vi "main(Test DQMH modules).vi"() -> ()   [LabVIEW 2018, in "Application.lvlib"] (continued)
        n2572 = Replace Array Subset(array=w5988, new element=w5987) -> (w5986:bool[])  [unwired: 1 in]
        n2573 = To Variant(anything=T3."mux10_1_channel3" ("mux10_1(x6)_encode")) -> (Variant=w6003:variant)
        n2574 = To Variant(anything=T4."demux1_10_channel3" ("demux1_10(x6)_encode")) -> (Variant=w5999:variant)
        n2575 = To Variant(anything=w5986) -> (Variant=w5995:variant)
        n2576 = Bundle By Name(cluster=w5992, "command"="MEAS.mux10-1", "data"=w6003) -> (w5998:T9)
        n2577 = Bundle By Name(cluster=w5992, "command"="MEAS.demux1-10", "data"=w5999) -> (w5997:T9)
        n2578 = Bundle By Name(cluster=w5992, "command"="MEAS.eMIC", "data"=w5995) -> (w5994:T9)
        n2579 = Build Array(w5998, w5997, w5994) -> (w6021:T9[])
        n2580 = Reverse 1D Array(array=w6021) -> (reversed array=w6020:T9[])
        n2581 = for {
          tunnel: w6020 -> [w6069] mode=indexing
          tunnel: [w6066] -> w6028 mode=indexing
          tunnel: w6022 -> [w6065]
          tunnel: w6025 -> [w6070]
          n2582 = Unbundle By Name(w6069) -> ("command"=w6068:string, "data"=w6067:variant)
          n2583 = call "App enquece.vi"("Priority Enquece"=TRUE, "error in (no error)"=w6065, "command data"=w6067, "command"=w6068, "queue in"=w6070) -> ("error out"=w6066:errorcluster)  [unwired: 5 in, 1 out]
        }
        n2584 = Merge Errors(w6031, w6028) -> (w6032:errorcluster)
      }
      frame "Test Channel 4D" {
        w6077 = T9 {"command"="", "data"=variant} ("element")
        w6098 = T9 {"command"="", "data"=variant} ("element")
        w6119 = 4  # DUT channel (1-10)
        n2585 = disable-structure shown="LOGGING==TRUE" {
          disable-tunnel: w6114 -> [w6146 _]
          frame condition #0 (active) {
            n2586 = Empty String/Path?(string/path=w6146) -> (empty?=w6148:bool)
            n2587 = Select(t="Quece timeout", s=w6148, f=w6146) -> (s? t:f=w6145:string)
            n2588 = call "string log (SubVI).vi"("state Name"=w6145) -> ()  [unwired: 9 in, 2 out]
          }
          frame condition #1 {
          }
        }
        n2589 = Bundle By Name(cluster=w6098, "command"="Apps.WaitForEvent") -> (w6096:T9)
        n2590 = Bundle By Name(cluster=w6098, "command"="Apps.UI Update", "data"="D") -> (w6097:T9)
        n2591 = Bundle By Name(cluster=w6098, "command"="MEAS.AllRelaysOFF2") -> (w6091:T9)
        n2592 = Build Array(w6097, w6091, w6096) -> (w6103:T9[])
        n2593 = for {
          tunnel: [w6136] -> w6109 mode=indexing
          shift-right: [w6137] -> w6111
          shift-left: w6104 -> [w6135]
          tunnel: w6103 -> [w6134] mode=indexing
          n2594 = Unbundle By Name(w6134) -> ("command"=w6133:string, "data"=w6132:variant)
          n2595 = call "App enquece.vi"("Priority Enquece"=TRUE, "command data"=w6132, "command"=w6133, "queue in"=w6135) -> ("error out"=w6136:errorcluster, "Queue out"=w6137:refnum<queue>)  [unwired: 6 in]
        }
        n2596 = call "FGV DRV stand.vi"() -> ("Sub-Test.DCV"=w6092:bool)  [unwired: 10 in, 1 out]
        n2597 = case shown="True" w6092 {
          tunnel: [w6122 w6131] -> w6112
          frame False {
            n2598 = Build Array("WaitFor", "MEAS.requestAC") -> (w6122:string[])
          }
          frame True {
            n2599 = Build Array("Test DRV 19", "Test DRV 20", "Test DRV 21", "Test DRV 22", "WaitForD", "MEAS.requestAC") -> (w6131:string[])
          }
        }
        n2600 = Merge Errors(w6109) -> (w6102:errorcluster)
        n2601 = Reverse 1D Array(array=w6112) -> (reversed array=w6090:string[])
        n2602 = for {
          tunnel: w6090 -> [w6143] mode=indexing
          tunnel: [w6142] -> w6108 mode=indexing
          shift-right: [w6141] -> w6110
          shift-left: w6111 -> [w6144]
          tunnel: w6102 -> [w6140]
          n2603 = call "App enquece.vi"("Priority Enquece"=TRUE, "error in (no error)"=w6140, "command"=w6143, "queue in"=w6144) -> ("error out"=w6142:errorcluster, "Queue out"=w6141:refnum<queue>)  [unwired: 6 in]
        }
        n2604 = Initialize Array(FALSE ("element"), 6 ("dimension size")) -> (w6073:bool[])
        n2605 = Initialize Array(TRUE, 4 ("dimension size")) -> (w6072:bool[])
        n2606 = Merge Errors(w6108) -> (w6107:errorcluster)
        n2607 = Replace Array Subset(array=w6073, new element=w6072) -> (w6071:bool[])  [unwired: 1 in]
        n2608 = To Variant(anything=T3."mux10_1_channel4" ("mux10_1(x6)_encode")) -> (Variant=w6088:variant)
        n2609 = To Variant(anything=T4."demux1_10_channel4" ("demux1_10(x6)_encode")) -> (Variant=w6084:variant)
        n2610 = To Variant(anything=w6071) -> (Variant=w6080:variant)
        n2611 = Bundle By Name(cluster=w6077, "command"="MEAS.mux10-1", "data"=w6088) -> (w6083:T9)
        n2612 = Bundle By Name(cluster=w6077, "command"="MEAS.demux1-10", "data"=w6084) -> (w6082:T9)
        n2613 = Bundle By Name(cluster=w6077, "command"="MEAS.eMIC", "data"=w6080) -> (w6079:T9)
        n2614 = Build Array(w6083, w6082, w6079) -> (w6106:T9[])
        n2615 = Reverse 1D Array(array=w6106) -> (reversed array=w6105:T9[])
        n2616 = for {
          tunnel: w6105 -> [w6154] mode=indexing
          tunnel: [w6151] -> w6113 mode=indexing
          tunnel: w6107 -> [w6150]
          tunnel: w6110 -> [w6155]
          n2617 = Unbundle By Name(w6154) -> ("command"=w6153:string, "data"=w6152:variant)
          n2618 = call "App enquece.vi"("Priority Enquece"=TRUE, "error in (no error)"=w6150, "command data"=w6152, "command"=w6153, "queue in"=w6155) -> ("error out"=w6151:errorcluster)  [unwired: 5 in, 1 out]
        }
        n2619 = Merge Errors(w6116, w6113) -> (w6117:errorcluster)
      }
      frame "Test Channel 5D" {
        w6162 = T9 {"command"="", "data"=variant} ("element")
        w6183 = T9 {"command"="", "data"=variant} ("element")
        w6204 = 5  # DUT channel (1-10)
        n2620 = disable-structure shown="LOGGING==TRUE" {
          disable-tunnel: w6199 -> [w6231 _]
          frame condition #0 (active) {
            n2621 = Empty String/Path?(string/path=w6231) -> (empty?=w6233:bool)
            n2622 = Select(t="Quece timeout", s=w6233, f=w6231) -> (s? t:f=w6230:string)
            n2623 = call "string log (SubVI).vi"("state Name"=w6230) -> ()  [unwired: 9 in, 2 out]
          }
          frame condition #1 {
          }
        }
        n2624 = Bundle By Name(cluster=w6183, "command"="Apps.UI Update", "data"="D") -> (w6182:T9)
        n2625 = Bundle By Name(cluster=w6183, "command"="MEAS.AllRelaysOFF2") -> (w6176:T9)
        n2626 = Bundle By Name(cluster=w6183, "command"="Apps.WaitForEvent") -> (w6181:T9)
        n2627 = Build Array(w6182, w6176, w6181) -> (w6188:T9[])
        n2628 = for {
          tunnel: [w6221] -> w6194 mode=indexing
          shift-right: [w6222] -> w6196
          shift-left: w6189 -> [w6220]
          tunnel: w6188 -> [w6219] mode=indexing
          n2629 = Unbundle By Name(w6219) -> ("command"=w6218:string, "data"=w6217:variant)
          n2630 = call "App enquece.vi"("Priority Enquece"=TRUE, "command data"=w6217, "command"=w6218, "queue in"=w6220) -> ("error out"=w6221:errorcluster, "Queue out"=w6222:refnum<queue>)  [unwired: 6 in]
        }
        n2631 = call "FGV DRV stand.vi"() -> ("Sub-Test.DCV"=w6177:bool)  [unwired: 10 in, 1 out]
        n2632 = case shown="True" w6177 {
          tunnel: [w6207 w6216] -> w6197
          frame False {
            n2633 = Build Array("WaitFor", "MEAS.requestAC") -> (w6207:string[])
          }
          frame True {
            n2634 = Build Array("Test DRV 25", "Test DRV 26", "Test DRV 27", "Test DRV 28", "WaitForD", "MEAS.requestAC") -> (w6216:string[])
          }
        }
        n2635 = Merge Errors(w6194) -> (w6187:errorcluster)
        n2636 = Reverse 1D Array(array=w6197) -> (reversed array=w6175:string[])
        n2637 = for {
          tunnel: w6175 -> [w6228] mode=indexing
          tunnel: [w6227] -> w6193 mode=indexing
          shift-right: [w6226] -> w6195
          shift-left: w6196 -> [w6229]
          tunnel: w6187 -> [w6225]
          n2638 = call "App enquece.vi"("Priority Enquece"=TRUE, "error in (no error)"=w6225, "command"=w6228, "queue in"=w6229) -> ("error out"=w6227:errorcluster, "Queue out"=w6226:refnum<queue>)  [unwired: 6 in]
        }
        n2639 = Merge Errors(w6193) -> (w6192:errorcluster)
        n2640 = Initialize Array(FALSE ("element"), 6 ("dimension size")) -> (w6158:bool[])
        n2641 = Initialize Array(TRUE, 4 ("dimension size")) -> (w6157:bool[])
        n2642 = Replace Array Subset(array=w6158, new element=w6157) -> (w6156:bool[])  [unwired: 1 in]
        n2643 = To Variant(anything=T3."mux10_1_channel5" ("mux10_1(x6)_encode")) -> (Variant=w6173:variant)
        n2644 = To Variant(anything=T4."demux1_10_channel5" ("demux1_10(x6)_encode")) -> (Variant=w6169:variant)
        n2645 = To Variant(anything=w6156) -> (Variant=w6165:variant)
        n2646 = Bundle By Name(cluster=w6162, "command"="MEAS.mux10-1", "data"=w6173) -> (w6168:T9)
        n2647 = Bundle By Name(cluster=w6162, "command"="MEAS.demux1-10", "data"=w6169) -> (w6167:T9)
        n2648 = Bundle By Name(cluster=w6162, "command"="MEAS.eMIC", "data"=w6165) -> (w6164:T9)
        n2649 = Build Array(w6168, w6167, w6164) -> (w6191:T9[])
        n2650 = Reverse 1D Array(array=w6191) -> (reversed array=w6190:T9[])
        n2651 = for {
          tunnel: w6190 -> [w6239] mode=indexing
          tunnel: [w6236] -> w6198 mode=indexing
          tunnel: w6192 -> [w6235]
          tunnel: w6195 -> [w6240]
          n2652 = Unbundle By Name(w6239) -> ("command"=w6238:string, "data"=w6237:variant)
          n2653 = call "App enquece.vi"("Priority Enquece"=TRUE, "error in (no error)"=w6235, "command data"=w6237, "command"=w6238, "queue in"=w6240) -> ("error out"=w6236:errorcluster)  [unwired: 5 in, 1 out]
        }
        n2654 = Merge Errors(w6201, w6198) -> (w6202:errorcluster)
      }
      frame "Test Channel 6D" {
        w6247 = T9 {"command"="", "data"=variant} ("element")
        w6268 = T9 {"command"="", "data"=variant} ("element")
        w6289 = 6  # DUT channel (1-10)
        n2655 = disable-structure shown="LOGGING==TRUE" {
          disable-tunnel: w6284 -> [w6316 _]
          frame condition #0 (active) {
            n2656 = Empty String/Path?(string/path=w6316) -> (empty?=w6318:bool)
            n2657 = Select(t="Quece timeout", s=w6318, f=w6316) -> (s? t:f=w6315:string)
            n2658 = call "string log (SubVI).vi"("state Name"=w6315) -> ()  [unwired: 9 in, 2 out]
          }
          frame condition #1 {
          }
        }
        n2659 = Bundle By Name(cluster=w6268, "command"="Apps.UI Update", "data"="D") -> (w6267:T9)
        n2660 = Bundle By Name(cluster=w6268, "command"="MEAS.AllRelaysOFF2") -> (w6261:T9)
        n2661 = Bundle By Name(cluster=w6268, "command"="Apps.WaitForEvent") -> (w6266:T9)
        n2662 = Build Array(w6267, w6261, w6266) -> (w6273:T9[])
        n2663 = for {
          tunnel: [w6306] -> w6279 mode=indexing
          shift-right: [w6307] -> w6281
          shift-left: w6274 -> [w6305]
          tunnel: w6273 -> [w6304] mode=indexing
          n2664 = Unbundle By Name(w6304) -> ("command"=w6303:string, "data"=w6302:variant)
          n2665 = call "App enquece.vi"("Priority Enquece"=TRUE, "command data"=w6302, "command"=w6303, "queue in"=w6305) -> ("error out"=w6306:errorcluster, "Queue out"=w6307:refnum<queue>)  [unwired: 6 in]
        }
        n2666 = call "FGV DRV stand.vi"() -> ("Sub-Test.DCV"=w6262:bool)  [unwired: 10 in, 1 out]
        n2667 = case shown="True" w6262 {
          tunnel: [w6292 w6301] -> w6282
          frame False {
            n2668 = Build Array("WaitFor", "MEAS.requestAC") -> (w6292:string[])
          }
          frame True {
            n2669 = Build Array("Test DRV 31", "Test DRV 32", "Test DRV 33", "Test DRV 34", "WaitForD", "MEAS.requestAC") -> (w6301:string[])
          }
        }
        n2670 = Merge Errors(w6279) -> (w6272:errorcluster)
        n2671 = Reverse 1D Array(array=w6282) -> (reversed array=w6260:string[])
        n2672 = for {
          tunnel: w6260 -> [w6313] mode=indexing
          tunnel: [w6312] -> w6278 mode=indexing
          shift-right: [w6311] -> w6280
          shift-left: w6281 -> [w6314]
          tunnel: w6272 -> [w6310]
          n2673 = call "App enquece.vi"("Priority Enquece"=TRUE, "error in (no error)"=w6310, "command"=w6313, "queue in"=w6314) -> ("error out"=w6312:errorcluster, "Queue out"=w6311:refnum<queue>)  [unwired: 6 in]
        }
        n2674 = Initialize Array(FALSE ("element"), 6 ("dimension size")) -> (w6243:bool[])
        n2675 = Initialize Array(TRUE, 4 ("dimension size")) -> (w6242:bool[])
        n2676 = Merge Errors(w6278) -> (w6277:errorcluster)
        n2677 = Replace Array Subset(array=w6243, new element=w6242) -> (w6241:bool[])  [unwired: 1 in]
        n2678 = To Variant(anything=T3."mux10_1_channel6" ("mux10_1(x6)_encode")) -> (Variant=w6258:variant)
        n2679 = To Variant(anything=T4."demux1_10_channel6" ("demux1_10(x6)_encode")) -> (Variant=w6254:variant)
        n2680 = To Variant(anything=w6241) -> (Variant=w6250:variant)
        n2681 = Bundle By Name(cluster=w6247, "command"="MEAS.mux10-1", "data"=w6258) -> (w6253:T9)
        n2682 = Bundle By Name(cluster=w6247, "command"="MEAS.demux1-10", "data"=w6254) -> (w6252:T9)
        n2683 = Bundle By Name(cluster=w6247, "command"="MEAS.eMIC", "data"=w6250) -> (w6249:T9)
        n2684 = Build Array(w6253, w6252, w6249) -> (w6276:T9[])
        n2685 = Reverse 1D Array(array=w6276) -> (reversed array=w6275:T9[])
        n2686 = for {
          tunnel: w6275 -> [w6324] mode=indexing
          tunnel: [w6321] -> w6283 mode=indexing
          tunnel: w6277 -> [w6320]
          tunnel: w6280 -> [w6325]
          n2687 = Unbundle By Name(w6324) -> ("command"=w6323:string, "data"=w6322:variant)
          n2688 = call "App enquece.vi"("Priority Enquece"=TRUE, "error in (no error)"=w6320, "command data"=w6322, "command"=w6323, "queue in"=w6325) -> ("error out"=w6321:errorcluster)  [unwired: 5 in, 1 out]
        }
        n2689 = Merge Errors(w6286, w6283) -> (w6287:errorcluster)
      }
      frame "Test Channel 7D" {
        w6332 = T9 {"command"="", "data"=variant} ("element")
        w6353 = T9 {"command"="", "data"=variant} ("element")
        w6374 = 7  # DUT channel (1-10)
        n2690 = disable-structure shown="LOGGING==TRUE" {
          disable-tunnel: w6369 -> [w6401 _]
          frame condition #0 (active) {
            n2691 = Empty String/Path?(string/path=w6401) -> (empty?=w6403:bool)
            n2692 = Select(t="Quece timeout", s=w6403, f=w6401) -> (s? t:f=w6400:string)
            n2693 = call "string log (SubVI).vi"("state Name"=w6400) -> ()  [unwired: 9 in, 2 out]
          }
          frame condition #1 {
          }
        }
        n2694 = Bundle By Name(cluster=w6353, "command"="Apps.UI Update", "data"="D") -> (w6352:T9)
        n2695 = Bundle By Name(cluster=w6353, "command"="MEAS.AllRelaysOFF2") -> (w6346:T9)
        n2696 = Bundle By Name(cluster=w6353, "command"="Apps.WaitForEvent") -> (w6351:T9)
        n2697 = Build Array(w6352, w6346, w6351) -> (w6358:T9[])
        n2698 = for {
          tunnel: [w6391] -> w6364 mode=indexing
          shift-right: [w6392] -> w6366
          shift-left: w6359 -> [w6390]
          tunnel: w6358 -> [w6389] mode=indexing
          n2699 = Unbundle By Name(w6389) -> ("command"=w6388:string, "data"=w6387:variant)
          n2700 = call "App enquece.vi"("Priority Enquece"=TRUE, "command data"=w6387, "command"=w6388, "queue in"=w6390) -> ("error out"=w6391:errorcluster, "Queue out"=w6392:refnum<queue>)  [unwired: 6 in]
        }
        n2701 = call "FGV DRV stand.vi"() -> ("Sub-Test.DCV"=w6347:bool)  [unwired: 10 in, 1 out]
        n2702 = case shown="True" w6347 {
          tunnel: [w6377 w6386] -> w6367
          frame False {
            n2703 = Build Array("WaitFor", "MEAS.requestAC") -> (w6377:string[])
          }
          frame True {
            n2704 = Build Array("Test DRV 37", "Test DRV 38", "Test DRV 39", "Test DRV 40", "WaitForD", "MEAS.requestAC") -> (w6386:string[])
          }
        }
        n2705 = Merge Errors(w6364) -> (w6357:errorcluster)
        n2706 = Reverse 1D Array(array=w6367) -> (reversed array=w6345:string[])
        n2707 = for {
          tunnel: w6345 -> [w6398] mode=indexing
          tunnel: [w6397] -> w6363 mode=indexing
          shift-right: [w6396] -> w6365
          shift-left: w6366 -> [w6399]
          tunnel: w6357 -> [w6395]
          n2708 = call "App enquece.vi"("Priority Enquece"=TRUE, "error in (no error)"=w6395, "command"=w6398, "queue in"=w6399) -> ("error out"=w6397:errorcluster, "Queue out"=w6396:refnum<queue>)  [unwired: 6 in]
        }
        n2709 = Initialize Array(FALSE ("element"), 6 ("dimension size")) -> (w6328:bool[])
        n2710 = Initialize Array(TRUE, 4 ("dimension size")) -> (w6327:bool[])
        n2711 = Merge Errors(w6363) -> (w6362:errorcluster)
        n2712 = Replace Array Subset(array=w6328, new element=w6327) -> (w6326:bool[])  [unwired: 1 in]
        n2713 = To Variant(anything=T3."mux10_1_channel7" ("mux10_1(x6)_encode")) -> (Variant=w6343:variant)
        n2714 = To Variant(anything=T4."demux1_10_channel7" ("demux1_10(x6)_encode")) -> (Variant=w6339:variant)
        n2715 = To Variant(anything=w6326) -> (Variant=w6335:variant)
        n2716 = Bundle By Name(cluster=w6332, "command"="MEAS.mux10-1", "data"=w6343) -> (w6338:T9)
        n2717 = Bundle By Name(cluster=w6332, "command"="MEAS.demux1-10", "data"=w6339) -> (w6337:T9)
        n2718 = Bundle By Name(cluster=w6332, "command"="MEAS.eMIC", "data"=w6335) -> (w6334:T9)
        n2719 = Build Array(w6338, w6337, w6334) -> (w6361:T9[])
        n2720 = Reverse 1D Array(array=w6361) -> (reversed array=w6360:T9[])
        n2721 = for {
          tunnel: w6360 -> [w6409] mode=indexing
          tunnel: [w6406] -> w6368 mode=indexing
          tunnel: w6362 -> [w6405]
          tunnel: w6365 -> [w6410]
          n2722 = Unbundle By Name(w6409) -> ("command"=w6408:string, "data"=w6407:variant)
          n2723 = call "App enquece.vi"("Priority Enquece"=TRUE, "error in (no error)"=w6405, "command data"=w6407, "command"=w6408, "queue in"=w6410) -> ("error out"=w6406:errorcluster)  [unwired: 5 in, 1 out]
        }
        n2724 = Merge Errors(w6371, w6368) -> (w6372:errorcluster)
      }
      frame "Test Channel 8D" {
        w6417 = T9 {"command"="", "data"=variant} ("element")
        w6438 = T9 {"command"="", "data"=variant} ("element")
        w6459 = 8  # DUT channel (1-10)
        n2725 = disable-structure shown="LOGGING==TRUE" {
          disable-tunnel: w6454 -> [w6486 _]
          frame condition #0 (active) {
            n2726 = Empty String/Path?(string/path=w6486) -> (empty?=w6488:bool)
            n2727 = Select(t="Quece timeout", s=w6488, f=w6486) -> (s? t:f=w6485:string)
            n2728 = call "string log (SubVI).vi"("state Name"=w6485) -> ()  [unwired: 9 in, 2 out]
          }
          frame condition #1 {
          }
        }
        n2729 = Bundle By Name(cluster=w6438, "command"="Apps.UI Update", "data"="D") -> (w6437:T9)
        n2730 = Bundle By Name(cluster=w6438, "command"="MEAS.AllRelaysOFF2") -> (w6431:T9)
        n2731 = Bundle By Name(cluster=w6438, "command"="Apps.WaitForEvent") -> (w6436:T9)
        n2732 = Build Array(w6437, w6431, w6436) -> (w6443:T9[])
        n2733 = for {
          tunnel: [w6476] -> w6449 mode=indexing
          shift-right: [w6477] -> w6451
          shift-left: w6444 -> [w6475]
          tunnel: w6443 -> [w6474] mode=indexing
          n2734 = Unbundle By Name(w6474) -> ("command"=w6473:string, "data"=w6472:variant)
          n2735 = call "App enquece.vi"("Priority Enquece"=TRUE, "command data"=w6472, "command"=w6473, "queue in"=w6475) -> ("error out"=w6476:errorcluster, "Queue out"=w6477:refnum<queue>)  [unwired: 6 in]
        }
        n2736 = call "FGV DRV stand.vi"() -> ("Sub-Test.DCV"=w6432:bool)  [unwired: 10 in, 1 out]
        n2737 = case shown="True" w6432 {
          tunnel: [w6462 w6471] -> w6452
          frame False {
            n2738 = Build Array("WaitFor", "MEAS.requestAC") -> (w6462:string[])
          }
          frame True {
            n2739 = Build Array("Test DRV 43", "Test DRV 44", "Test DRV 45", "Test DRV 46", "WaitForD", "MEAS.requestAC") -> (w6471:string[])
          }
        }
        n2740 = Merge Errors(w6449) -> (w6442:errorcluster)
        n2741 = Reverse 1D Array(array=w6452) -> (reversed array=w6430:string[])
        n2742 = for {
          tunnel: w6430 -> [w6483] mode=indexing
          tunnel: [w6482] -> w6448 mode=indexing
          shift-right: [w6481] -> w6450
          shift-left: w6451 -> [w6484]
          tunnel: w6442 -> [w6480]
          n2743 = call "App enquece.vi"("Priority Enquece"=TRUE, "error in (no error)"=w6480, "command"=w6483, "queue in"=w6484) -> ("error out"=w6482:errorcluster, "Queue out"=w6481:refnum<queue>)  [unwired: 6 in]
        }
        n2744 = Initialize Array(FALSE ("element"), 6 ("dimension size")) -> (w6413:bool[])
        n2745 = Initialize Array(TRUE, 4 ("dimension size")) -> (w6412:bool[])
        n2746 = Merge Errors(w6448) -> (w6447:errorcluster)
        n2747 = Replace Array Subset(array=w6413, new element=w6412) -> (w6411:bool[])  [unwired: 1 in]
        n2748 = To Variant(anything=T3."mux10_1_channel8" ("mux10_1(x6)_encode")) -> (Variant=w6428:variant)
        n2749 = To Variant(anything=T4."demux1_10_channel8" ("demux1_10(x6)_encode")) -> (Variant=w6424:variant)
        n2750 = To Variant(anything=w6411) -> (Variant=w6420:variant)
        n2751 = Bundle By Name(cluster=w6417, "command"="MEAS.mux10-1", "data"=w6428) -> (w6423:T9)
        n2752 = Bundle By Name(cluster=w6417, "command"="MEAS.demux1-10", "data"=w6424) -> (w6422:T9)
        n2753 = Bundle By Name(cluster=w6417, "command"="MEAS.eMIC", "data"=w6420) -> (w6419:T9)
        n2754 = Build Array(w6423, w6422, w6419) -> (w6446:T9[])
        n2755 = Reverse 1D Array(array=w6446) -> (reversed array=w6445:T9[])
        n2756 = for {
          tunnel: w6445 -> [w6494] mode=indexing
          tunnel: [w6491] -> w6453 mode=indexing
          tunnel: w6447 -> [w6490]
          tunnel: w6450 -> [w6495]
          n2757 = Unbundle By Name(w6494) -> ("command"=w6493:string, "data"=w6492:variant)
          n2758 = call "App enquece.vi"("Priority Enquece"=TRUE, "error in (no error)"=w6490, "command data"=w6492, "command"=w6493, "queue in"=w6495) -> ("error out"=w6491:errorcluster)  [unwired: 5 in, 1 out]
        }
        n2759 = Merge Errors(w6456, w6453) -> (w6457:errorcluster)
      }
      frame "Test Channel 9D" {
        w6502 = T9 {"command"="", "data"=variant} ("element")
        w6523 = T9 {"command"="", "data"=variant} ("element")
        w6544 = 9  # DUT channel (1-10)
        n2760 = disable-structure shown="LOGGING==TRUE" {
          disable-tunnel: w6539 -> [w6571 _]
          frame condition #0 (active) {
            n2761 = Empty String/Path?(string/path=w6571) -> (empty?=w6573:bool)
            n2762 = Select(t="Quece timeout", s=w6573, f=w6571) -> (s? t:f=w6570:string)
            n2763 = call "string log (SubVI).vi"("state Name"=w6570) -> ()  [unwired: 9 in, 2 out]
          }
          frame condition #1 {
          }
        }
        n2764 = Bundle By Name(cluster=w6523, "command"="Apps.UI Update", "data"="D") -> (w6522:T9)
        n2765 = Bundle By Name(cluster=w6523, "command"="MEAS.AllRelaysOFF2") -> (w6516:T9)
        n2766 = Bundle By Name(cluster=w6523, "command"="Apps.WaitForEvent") -> (w6521:T9)
        n2767 = Build Array(w6522, w6516, w6521) -> (w6528:T9[])
        n2768 = for {
          tunnel: [w6561] -> w6534 mode=indexing
          shift-right: [w6562] -> w6536
          shift-left: w6529 -> [w6560]
          tunnel: w6528 -> [w6559] mode=indexing
          n2769 = Unbundle By Name(w6559) -> ("command"=w6558:string, "data"=w6557:variant)
          n2770 = call "App enquece.vi"("Priority Enquece"=TRUE, "command data"=w6557, "command"=w6558, "queue in"=w6560) -> ("error out"=w6561:errorcluster, "Queue out"=w6562:refnum<queue>)  [unwired: 6 in]
        }
        n2771 = call "FGV DRV stand.vi"() -> ("Sub-Test.DCV"=w6517:bool)  [unwired: 10 in, 1 out]
        n2772 = case shown="False" w6517 {
          tunnel: [w6547 w6556] -> w6537
          frame False {
            n2773 = Build Array("WaitFor", "MEAS.requestAC") -> (w6547:string[])
          }
          frame True {
            n2774 = Build Array("Test DRV 49", "Test DRV 50", "Test DRV 51", "Test DRV 52", "WaitForD", "MEAS.requestAC") -> (w6556:string[])
          }
        }
        n2775 = Merge Errors(w6534) -> (w6527:errorcluster)
        n2776 = Reverse 1D Array(array=w6537) -> (reversed array=w6515:string[])
        n2777 = for {
          tunnel: w6515 -> [w6568] mode=indexing
          tunnel: [w6567] -> w6533 mode=indexing
          shift-right: [w6566] -> w6535
          shift-left: w6536 -> [w6569]
          tunnel: w6527 -> [w6565]
          n2778 = call "App enquece.vi"("Priority Enquece"=TRUE, "error in (no error)"=w6565, "command"=w6568, "queue in"=w6569) -> ("error out"=w6567:errorcluster, "Queue out"=w6566:refnum<queue>)  [unwired: 6 in]
        }
        n2779 = Initialize Array(FALSE ("element"), 6 ("dimension size")) -> (w6498:bool[])
        n2780 = Initialize Array(TRUE, 4 ("dimension size")) -> (w6497:bool[])
        n2781 = Merge Errors(w6533) -> (w6532:errorcluster)
        n2782 = Replace Array Subset(array=w6498, new element=w6497) -> (w6496:bool[])  [unwired: 1 in]
        n2783 = To Variant(anything=T3."mux10_1_channel9" ("mux10_1(x6)_encode")) -> (Variant=w6513:variant)
        n2784 = To Variant(anything=T4."demux1_10_channel9" ("demux1_10(x6)_encode")) -> (Variant=w6509:variant)
        n2785 = To Variant(anything=w6496) -> (Variant=w6505:variant)
        n2786 = Bundle By Name(cluster=w6502, "command"="MEAS.mux10-1", "data"=w6513) -> (w6508:T9)
        n2787 = Bundle By Name(cluster=w6502, "command"="MEAS.demux1-10", "data"=w6509) -> (w6507:T9)
        n2788 = Bundle By Name(cluster=w6502, "command"="MEAS.eMIC", "data"=w6505) -> (w6504:T9)
        n2789 = Build Array(w6508, w6507, w6504) -> (w6531:T9[])
        n2790 = Reverse 1D Array(array=w6531) -> (reversed array=w6530:T9[])
        n2791 = for {
          tunnel: w6530 -> [w6579] mode=indexing
          tunnel: [w6576] -> w6538 mode=indexing
          tunnel: w6532 -> [w6575]
          tunnel: w6535 -> [w6580]
          n2792 = Unbundle By Name(w6579) -> ("command"=w6578:string, "data"=w6577:variant)
          n2793 = call "App enquece.vi"("Priority Enquece"=TRUE, "error in (no error)"=w6575, "command data"=w6577, "command"=w6578, "queue in"=w6580) -> ("error out"=w6576:errorcluster)  [unwired: 5 in, 1 out]
        }
        n2794 = Merge Errors(w6541, w6538) -> (w6542:errorcluster)
      }
      frame "Test Channel 10E" {
        w6587 = T9 {"command"="", "data"=variant} ("element")
        w6609 = T9 {"command"="", "data"=variant} ("element")
        w6629 = 10  # DUT channel (1-10)
        n2795 = disable-structure shown="LOGGING==TRUE" {
          disable-tunnel: w6624 -> [w6657 _]
          frame condition #0 (active) {
            n2796 = Empty String/Path?(string/path=w6657) -> (empty?=w6659:bool)
            n2797 = Select(t="Quece timeout", s=w6659, f=w6657) -> (s? t:f=w6656:string)
            n2798 = call "string log (SubVI).vi"("state Name"=w6656) -> ()  [unwired: 9 in, 2 out]
          }
          frame condition #1 {
          }
        }
        n2799 = Bundle By Name(cluster=w6609, "command"="Apps.UI Update", "data"="E") -> (w6608:T9)
        n2800 = Bundle By Name(cluster=w6609, "command"="MEAS.AllRelaysOFF2") -> (w6601:T9)
        n2801 = Bundle By Name(cluster=w6609, "command"="Apps.WaitForEvent") -> (w6607:T9)
        n2802 = Build Array(w6608, w6601, w6607) -> (w6614:T9[])
        n2803 = for {
          tunnel: [w6647] -> w6620 mode=indexing
          shift-right: [w6648] -> w6622
          shift-left: w6615 -> [w6646]
          tunnel: w6614 -> [w6645] mode=indexing
          n2804 = Unbundle By Name(w6645) -> ("command"=w6644:string, "data"=w6643:variant)
          n2805 = call "App enquece.vi"("Priority Enquece"=TRUE, "command data"=w6643, "command"=w6644, "queue in"=w6646) -> ("error out"=w6647:errorcluster, "Queue out"=w6648:refnum<queue>)  [unwired: 6 in]
        }
        n2806 = call "FGV DRV stand.vi"() -> ("Sub-Test.DCV"=w6602:bool)  [unwired: 10 in, 1 out]
        n2807 = case shown="True" w6602 {
          tunnel: [w6633 w6635] -> w6604
          frame False {
            n2808 = Build Array("WaitFor", "MEAS.requestAC") -> (w6633:string[])
          }
          frame True {
            n2809 = Build Array("Test DRV 55", "Test DRV 56", "Test DRV 57", "Test DRV 58", "Test DRV 59", "WaitForE", "MEAS.requestAC") -> (w6635:string[])
          }
        }
        n2810 = Merge Errors(w6620) -> (w6613:errorcluster)
        n2811 = Reverse 1D Array(array=w6604) -> (reversed array=w6600:string[])
        n2812 = for {
          tunnel: w6600 -> [w6654] mode=indexing
          tunnel: [w6653] -> w6619 mode=indexing
          shift-right: [w6652] -> w6621
          shift-left: w6622 -> [w6655]
          tunnel: w6613 -> [w6651]
          n2813 = call "App enquece.vi"("Priority Enquece"=TRUE, "error in (no error)"=w6651, "command"=w6654, "queue in"=w6655) -> ("error out"=w6653:errorcluster, "Queue out"=w6652:refnum<queue>)  [unwired: 6 in]
        }
        n2814 = Initialize Array(FALSE ("element"), 6 ("dimension size")) -> (w6583:bool[])
        n2815 = Initialize Array(TRUE, 5 ("dimension size")) -> (w6582:bool[])
        n2816 = Merge Errors(w6619) -> (w6618:errorcluster)
        n2817 = Replace Array Subset(array=w6583, new element=w6582) -> (w6581:bool[])  [unwired: 1 in]
        n2818 = To Variant(anything=T3."mux10_1_channel10" ("mux10_1(x6)_encode")) -> (Variant=w6598:variant)
        n2819 = To Variant(anything=T4."demux1_10_channel10" ("demux1_10(x6)_encode")) -> (Variant=w6594:variant)
        n2820 = To Variant(anything=w6581) -> (Variant=w6590:variant)
        n2821 = Bundle By Name(cluster=w6587, "command"="MEAS.mux10-1", "data"=w6598) -> (w6593:T9)
        n2822 = Bundle By Name(cluster=w6587, "command"="MEAS.demux1-10", "data"=w6594) -> (w6592:T9)
        n2823 = Bundle By Name(cluster=w6587, "command"="MEAS.eMIC", "data"=w6590) -> (w6589:T9)
        n2824 = Build Array(w6593, w6592, w6589) -> (w6617:T9[])
        n2825 = Reverse 1D Array(array=w6617) -> (reversed array=w6616:T9[])
        n2826 = for {
          tunnel: w6616 -> [w6665] mode=indexing
          tunnel: [w6662] -> w6623 mode=indexing
          tunnel: w6618 -> [w6661]
          tunnel: w6621 -> [w6666]
          n2827 = Unbundle By Name(w6665) -> ("command"=w6664:string, "data"=w6663:variant)
          n2828 = call "App enquece.vi"("Priority Enquece"=TRUE, "error in (no error)"=w6661, "command data"=w6663, "command"=w6664, "queue in"=w6666) -> ("error out"=w6662:errorcluster)  [unwired: 5 in, 1 out]
        }
        n2829 = Merge Errors(w6626, w6623) -> (w6627:errorcluster)
      }
      frame "Test Channel 1E" {
        w6673 = T9 {"command"="", "data"=variant} ("element")
        w6695 = T9 {"command"="", "data"=variant} ("element")
        w6715 = 1  # DUT channel (1-10)
        n2830 = disable-structure shown="LOGGING==TRUE" {
          disable-tunnel: w6710 -> [w6743 _]
          frame condition #0 (active) {
            n2831 = Empty String/Path?(string/path=w6743) -> (empty?=w6745:bool)
            n2832 = Select(t="Quece timeout", s=w6745, f=w6743) -> (s? t:f=w6742:string)
            n2833 = call "string log (SubVI).vi"("state Name"=w6742) -> ()  [unwired: 9 in, 2 out]
          }
          frame condition #1 {
          }
        }
        n2834 = Bundle By Name(cluster=w6695, "command"="Apps.UI Update", "data"="E") -> (w6694:T9)
        n2835 = Bundle By Name(cluster=w6695, "command"="MEAS.AllRelaysOFF2") -> (w6687:T9)
        n2836 = Bundle By Name(cluster=w6695, "command"="Apps.WaitForEvent") -> (w6693:T9)
        n2837 = Build Array(w6694, w6687, w6693) -> (w6700:T9[])
        n2838 = for {
          tunnel: [w6733] -> w6706 mode=indexing
          shift-right: [w6734] -> w6708
          shift-left: w6701 -> [w6732]
          tunnel: w6700 -> [w6731] mode=indexing
          n2839 = Unbundle By Name(w6731) -> ("command"=w6730:string, "data"=w6729:variant)
          n2840 = call "App enquece.vi"("Priority Enquece"=TRUE, "command data"=w6729, "command"=w6730, "queue in"=w6732) -> ("error out"=w6733:errorcluster, "Queue out"=w6734:refnum<queue>)  [unwired: 6 in]
        }
        n2841 = call "FGV DRV stand.vi"() -> ("Sub-Test.DCV"=w6688:bool)  [unwired: 10 in, 1 out]
        n2842 = case shown="True" w6688 {
          tunnel: [w6719 w6721] -> w6690
          frame False {
            n2843 = Build Array("WaitFor", "MEAS.requestAC") -> (w6719:string[])
          }
          frame True {
            n2844 = Build Array("Test DRV 1", "Test DRV 2", "Test DRV 3", "Test DRV 4", "Test DRV 5", "WaitForE", "MEAS.requestAC") -> (w6721:string[])
          }
        }
        n2845 = Merge Errors(w6706) -> (w6699:errorcluster)
        n2846 = Reverse 1D Array(array=w6690) -> (reversed array=w6686:string[])
        n2847 = for {
          tunnel: w6686 -> [w6740] mode=indexing
          tunnel: [w6739] -> w6705 mode=indexing
          shift-right: [w6738] -> w6707
          shift-left: w6708 -> [w6741]
          tunnel: w6699 -> [w6737]
          n2848 = call "App enquece.vi"("Priority Enquece"=TRUE, "error in (no error)"=w6737, "command"=w6740, "queue in"=w6741) -> ("error out"=w6739:errorcluster, "Queue out"=w6738:refnum<queue>)  [unwired: 6 in]
        }
        n2849 = Initialize Array(FALSE ("element"), 6 ("dimension size")) -> (w6669:bool[])
        n2850 = Initialize Array(TRUE, 5 ("dimension size")) -> (w6668:bool[])
        n2851 = Merge Errors(w6705) -> (w6704:errorcluster)
        n2852 = Replace Array Subset(array=w6669, new element=w6668) -> (w6667:bool[])  [unwired: 1 in]
        n2853 = To Variant(anything=T3."mux10_1_channel1" ("mux10_1(x6)_encode")) -> (Variant=w6684:variant)
        n2854 = To Variant(anything=T4."demux1_10_channel1" ("demux1_10(x6)_encode")) -> (Variant=w6680:variant)
        n2855 = To Variant(anything=w6667) -> (Variant=w6676:variant)
        n2856 = Bundle By Name(cluster=w6673, "command"="MEAS.mux10-1", "data"=w6684) -> (w6679:T9)
        n2857 = Bundle By Name(cluster=w6673, "command"="MEAS.demux1-10", "data"=w6680) -> (w6678:T9)
        n2858 = Bundle By Name(cluster=w6673, "command"="MEAS.eMIC", "data"=w6676) -> (w6675:T9)
        n2859 = Build Array(w6679, w6678, w6675) -> (w6703:T9[])
        n2860 = Reverse 1D Array(array=w6703) -> (reversed array=w6702:T9[])
        n2861 = for {
          tunnel: w6702 -> [w6751] mode=indexing
          tunnel: [w6748] -> w6709 mode=indexing
          tunnel: w6704 -> [w6747]
          tunnel: w6707 -> [w6752]
          n2862 = Unbundle By Name(w6751) -> ("command"=w6750:string, "data"=w6749:variant)
          n2863 = call "App enquece.vi"("Priority Enquece"=TRUE, "error in (no error)"=w6747, "command data"=w6749, "command"=w6750, "queue in"=w6752) -> ("error out"=w6748:errorcluster)  [unwired: 5 in, 1 out]
        }
        n2864 = Merge Errors(w6712, w6709) -> (w6713:errorcluster)
      }
      frame "Test Channel 2E" {
        w6759 = T9 {"command"="", "data"=variant} ("element")
        w6781 = T9 {"command"="", "data"=variant} ("element")
        w6801 = 2  # DUT channel (1-10)
        n2865 = disable-structure shown="LOGGING==TRUE" {
          disable-tunnel: w6796 -> [w6829 _]
          frame condition #0 (active) {
            n2866 = Empty String/Path?(string/path=w6829) -> (empty?=w6831:bool)
            n2867 = Select(t="Quece timeout", s=w6831, f=w6829) -> (s? t:f=w6828:string)
            n2868 = call "string log (SubVI).vi"("state Name"=w6828) -> ()  [unwired: 9 in, 2 out]
          }
          frame condition #1 {
          }
        }
        n2869 = Bundle By Name(cluster=w6781, "command"="Apps.UI Update", "data"="E") -> (w6780:T9)
        n2870 = Bundle By Name(cluster=w6781, "command"="MEAS.AllRelaysOFF2") -> (w6773:T9)
        n2871 = Bundle By Name(cluster=w6781, "command"="Apps.WaitForEvent") -> (w6779:T9)
        n2872 = Build Array(w6780, w6773, w6779) -> (w6786:T9[])
        n2873 = for {
          tunnel: [w6819] -> w6792 mode=indexing
          shift-right: [w6820] -> w6794
          shift-left: w6787 -> [w6818]
          tunnel: w6786 -> [w6817] mode=indexing
          n2874 = Unbundle By Name(w6817) -> ("command"=w6816:string, "data"=w6815:variant)
          n2875 = call "App enquece.vi"("Priority Enquece"=TRUE, "command data"=w6815, "command"=w6816, "queue in"=w6818) -> ("error out"=w6819:errorcluster, "Queue out"=w6820:refnum<queue>)  [unwired: 6 in]
        }
        n2876 = call "FGV DRV stand.vi"() -> ("Sub-Test.DCV"=w6774:bool)  [unwired: 10 in, 1 out]
        n2877 = case shown="True" w6774 {
          tunnel: [w6805 w6807] -> w6776
          frame False {
            n2878 = Build Array("WaitFor", "MEAS.requestAC") -> (w6805:string[])
          }
          frame True {
            n2879 = Build Array("Test DRV 7", "Test DRV 8", "Test DRV 9", "Test DRV 10", "Test DRV 11", "WaitForE", "MEAS.requestAC") -> (w6807:string[])
          }
        }
        n2880 = Merge Errors(w6792) -> (w6785:errorcluster)
        n2881 = Reverse 1D Array(array=w6776) -> (reversed array=w6772:string[])
        n2882 = for {
          tunnel: w6772 -> [w6826] mode=indexing
          tunnel: [w6825] -> w6791 mode=indexing
          shift-right: [w6824] -> w6793
          shift-left: w6794 -> [w6827]
          tunnel: w6785 -> [w6823]
          n2883 = call "App enquece.vi"("Priority Enquece"=TRUE, "error in (no error)"=w6823, "command"=w6826, "queue in"=w6827) -> ("error out"=w6825:errorcluster, "Queue out"=w6824:refnum<queue>)  [unwired: 6 in]
        }
        n2884 = Initialize Array(FALSE ("element"), 6 ("dimension size")) -> (w6755:bool[])
        n2885 = Initialize Array(TRUE, 5 ("dimension size")) -> (w6754:bool[])
        n2886 = Merge Errors(w6791) -> (w6790:errorcluster)
        n2887 = Replace Array Subset(array=w6755, new element=w6754) -> (w6753:bool[])  [unwired: 1 in]
        n2888 = To Variant(anything=w6753) -> (Variant=w6762:variant)
        n2889 = To Variant(anything=T3."mux10_1_channel2" ("mux10_1(x6)_encode")) -> (Variant=w6770:variant)
        n2890 = To Variant(anything=T4."demux1_10_channel2" ("demux1_10(x6)_encode")) -> (Variant=w6766:variant)
        n2891 = Bundle By Name(cluster=w6759, "command"="MEAS.mux10-1", "data"=w6770) -> (w6765:T9)
        n2892 = Bundle By Name(cluster=w6759, "command"="MEAS.demux1-10", "data"=w6766) -> (w6764:T9)
        n2893 = Bundle By Name(cluster=w6759, "command"="MEAS.eMIC", "data"=w6762) -> (w6761:T9)
        n2894 = Build Array(w6765, w6764, w6761) -> (w6789:T9[])
        n2895 = Reverse 1D Array(array=w6789) -> (reversed array=w6788:T9[])
        n2896 = for {
          tunnel: w6788 -> [w6837] mode=indexing
          tunnel: [w6834] -> w6795 mode=indexing
          tunnel: w6790 -> [w6833]
          tunnel: w6793 -> [w6838]
          n2897 = Unbundle By Name(w6837) -> ("command"=w6836:string, "data"=w6835:variant)
          n2898 = call "App enquece.vi"("Priority Enquece"=TRUE, "error in (no error)"=w6833, "command data"=w6835, "command"=w6836, "queue in"=w6838) -> ("error out"=w6834:errorcluster)  [unwired: 5 in, 1 out]
        }
        n2899 = Merge Errors(w6798, w6795) -> (w6799:errorcluster)
      }
      frame "Test Channel 3E" {
        w6845 = T9 {"command"="", "data"=variant} ("element")
        w6867 = T9 {"command"="", "data"=variant} ("element")
        w6887 = 3  # DUT channel (1-10)
        n2900 = disable-structure shown="LOGGING==TRUE" {
          disable-tunnel: w6882 -> [w6915 _]
          frame condition #0 (active) {
            n2901 = Empty String/Path?(string/path=w6915) -> (empty?=w6917:bool)
            n2902 = Select(t="Quece timeout", s=w6917, f=w6915) -> (s? t:f=w6914:string)
            n2903 = call "string log (SubVI).vi"("state Name"=w6914) -> ()  [unwired: 9 in, 2 out]
          }
          frame condition #1 {
          }
        }
        n2904 = Bundle By Name(cluster=w6867, "command"="Apps.UI Update", "data"="E") -> (w6866:T9)
        n2905 = Bundle By Name(cluster=w6867, "command"="MEAS.AllRelaysOFF2") -> (w6859:T9)
        n2906 = Bundle By Name(cluster=w6867, "command"="Apps.WaitForEvent") -> (w6865:T9)
        n2907 = Build Array(w6866, w6859, w6865) -> (w6872:T9[])
        n2908 = for {
          tunnel: [w6905] -> w6878 mode=indexing
          shift-right: [w6906] -> w6880
          shift-left: w6873 -> [w6904]
          tunnel: w6872 -> [w6903] mode=indexing
          n2909 = Unbundle By Name(w6903) -> ("command"=w6902:string, "data"=w6901:variant)
          n2910 = call "App enquece.vi"("Priority Enquece"=TRUE, "command data"=w6901, "command"=w6902, "queue in"=w6904) -> ("error out"=w6905:errorcluster, "Queue out"=w6906:refnum<queue>)  [unwired: 6 in]
        }
        n2911 = call "FGV DRV stand.vi"() -> ("Sub-Test.DCV"=w6860:bool)  [unwired: 10 in, 1 out]
        n2912 = case shown="True" w6860 {
          tunnel: [w6891 w6893] -> w6862
          frame False {
            n2913 = Build Array("WaitFor", "MEAS.requestAC") -> (w6891:string[])
          }
          frame True {
            n2914 = Build Array("Test DRV 13", "Test DRV 14", "Test DRV 15", "Test DRV 16", "Test DRV 17", "WaitForE", "MEAS.requestAC") -> (w6893:string[])
          }
        }
        n2915 = Merge Errors(w6878) -> (w6871:errorcluster)
        n2916 = Reverse 1D Array(array=w6862) -> (reversed array=w6858:string[])
        n2917 = for {
          tunnel: w6858 -> [w6912] mode=indexing
          tunnel: [w6911] -> w6877 mode=indexing
          shift-right: [w6910] -> w6879
          shift-left: w6880 -> [w6913]
          tunnel: w6871 -> [w6909]
          n2918 = call "App enquece.vi"("Priority Enquece"=TRUE, "error in (no error)"=w6909, "command"=w6912, "queue in"=w6913) -> ("error out"=w6911:errorcluster, "Queue out"=w6910:refnum<queue>)  [unwired: 6 in]
        }
        n2919 = Initialize Array(FALSE ("element"), 6 ("dimension size")) -> (w6841:bool[])
        n2920 = Initialize Array(TRUE, 5 ("dimension size")) -> (w6840:bool[])
        n2921 = Replace Array Subset(array=w6841, new element=w6840) -> (w6839:bool[])  [unwired: 1 in]
        n2922 = Merge Errors(w6877) -> (w6876:errorcluster)
        n2923 = To Variant(anything=T3."mux10_1_channel3" ("mux10_1(x6)_encode")) -> (Variant=w6856:variant)
        n2924 = To Variant(anything=T4."demux1_10_channel3" ("demux1_10(x6)_encode")) -> (Variant=w6852:variant)
        n2925 = To Variant(anything=w6839) -> (Variant=w6848:variant)
        n2926 = Bundle By Name(cluster=w6845, "command"="MEAS.mux10-1", "data"=w6856) -> (w6851:T9)
        n2927 = Bundle By Name(cluster=w6845, "command"="MEAS.demux1-10", "data"=w6852) -> (w6850:T9)
        n2928 = Bundle By Name(cluster=w6845, "command"="MEAS.eMIC", "data"=w6848) -> (w6847:T9)
        n2929 = Build Array(w6851, w6850, w6847) -> (w6875:T9[])
        n2930 = Reverse 1D Array(array=w6875) -> (reversed array=w6874:T9[])
        n2931 = for {
          tunnel: w6874 -> [w6923] mode=indexing
          tunnel: [w6920] -> w6881 mode=indexing
          tunnel: w6876 -> [w6919]
          tunnel: w6879 -> [w6924]
          n2932 = Unbundle By Name(w6923) -> ("command"=w6922:string, "data"=w6921:variant)
          n2933 = call "App enquece.vi"("Priority Enquece"=TRUE, "error in (no error)"=w6919, "command data"=w6921, "command"=w6922, "queue in"=w6924) -> ("error out"=w6920:errorcluster)  [unwired: 5 in, 1 out]
        }
        n2934 = Merge Errors(w6884, w6881) -> (w6885:errorcluster)
      }
      frame "Test Channel 4E" {
        w6931 = T9 {"command"="", "data"=variant} ("element")
        w6953 = T9 {"command"="", "data"=variant} ("element")
        w6973 = 4  # DUT channel (1-10)
        n2935 = disable-structure shown="LOGGING==TRUE" {
          disable-tunnel: w6968 -> [w7001 _]
          frame condition #0 (active) {
            n2936 = Empty String/Path?(string/path=w7001) -> (empty?=w7003:bool)
            n2937 = Select(t="Quece timeout", s=w7003, f=w7001) -> (s? t:f=w7000:string)
            n2938 = call "string log (SubVI).vi"("state Name"=w7000) -> ()  [unwired: 9 in, 2 out]
          }
          frame condition #1 {
          }
        }
        n2939 = Bundle By Name(cluster=w6953, "command"="Apps.UI Update", "data"="E") -> (w6952:T9)
        n2940 = Bundle By Name(cluster=w6953, "command"="MEAS.AllRelaysOFF2") -> (w6945:T9)
        n2941 = Bundle By Name(cluster=w6953, "command"="Apps.WaitForEvent") -> (w6951:T9)
        n2942 = Build Array(w6952, w6945, w6951) -> (w6958:T9[])
        n2943 = for {
          tunnel: [w6991] -> w6964 mode=indexing
          shift-right: [w6992] -> w6966
          shift-left: w6959 -> [w6990]
          tunnel: w6958 -> [w6989] mode=indexing
          n2944 = Unbundle By Name(w6989) -> ("command"=w6988:string, "data"=w6987:variant)
          n2945 = call "App enquece.vi"("Priority Enquece"=TRUE, "command data"=w6987, "command"=w6988, "queue in"=w6990) -> ("error out"=w6991:errorcluster, "Queue out"=w6992:refnum<queue>)  [unwired: 6 in]
        }
        n2946 = call "FGV DRV stand.vi"() -> ("Sub-Test.DCV"=w6946:bool)  [unwired: 10 in, 1 out]
        n2947 = case shown="True" w6946 {
          tunnel: [w6977 w6979] -> w6948
          frame False {
            n2948 = Build Array("WaitFor", "MEAS.requestAC") -> (w6977:string[])
          }
          frame True {
            n2949 = Build Array("Test DRV 19", "Test DRV 20", "Test DRV 21", "Test DRV 22", "Test DRV 23", "WaitForE", "MEAS.requestAC") -> (w6979:string[])
          }
        }
        n2950 = Merge Errors(w6964) -> (w6957:errorcluster)
        n2951 = Reverse 1D Array(array=w6948) -> (reversed array=w6944:string[])
        n2952 = for {
          tunnel: w6944 -> [w6998] mode=indexing
          tunnel: [w6997] -> w6963 mode=indexing
          shift-right: [w6996] -> w6965
          shift-left: w6966 -> [w6999]
          tunnel: w6957 -> [w6995]
          n2953 = call "App enquece.vi"("Priority Enquece"=TRUE, "error in (no error)"=w6995, "command"=w6998, "queue in"=w6999) -> ("error out"=w6997:errorcluster, "Queue out"=w6996:refnum<queue>)  [unwired: 6 in]
        }
        n2954 = Initialize Array(FALSE ("element"), 6 ("dimension size")) -> (w6927:bool[])
        n2955 = Initialize Array(TRUE, 5 ("dimension size")) -> (w6926:bool[])
        n2956 = Merge Errors(w6963) -> (w6962:errorcluster)
        n2957 = Replace Array Subset(array=w6927, new element=w6926) -> (w6925:bool[])  [unwired: 1 in]
        n2958 = To Variant(anything=T3."mux10_1_channel4" ("mux10_1(x6)_encode")) -> (Variant=w6942:variant)
        n2959 = To Variant(anything=T4."demux1_10_channel4" ("demux1_10(x6)_encode")) -> (Variant=w6938:variant)
        n2960 = To Variant(anything=w6925) -> (Variant=w6934:variant)
        n2961 = Bundle By Name(cluster=w6931, "command"="MEAS.mux10-1", "data"=w6942) -> (w6937:T9)
        n2962 = Bundle By Name(cluster=w6931, "command"="MEAS.demux1-10", "data"=w6938) -> (w6936:T9)
        n2963 = Bundle By Name(cluster=w6931, "command"="MEAS.eMIC", "data"=w6934) -> (w6933:T9)
        n2964 = Build Array(w6937, w6936, w6933) -> (w6961:T9[])
        n2965 = Reverse 1D Array(array=w6961) -> (reversed array=w6960:T9[])
        n2966 = for {
          tunnel: w6960 -> [w7009] mode=indexing
          tunnel: [w7006] -> w6967 mode=indexing
          tunnel: w6962 -> [w7005]
          tunnel: w6965 -> [w7010]
          n2967 = Unbundle By Name(w7009) -> ("command"=w7008:string, "data"=w7007:variant)
          n2968 = call "App enquece.vi"("Priority Enquece"=TRUE, "error in (no error)"=w7005, "command data"=w7007, "command"=w7008, "queue in"=w7010) -> ("error out"=w7006:errorcluster)  [unwired: 5 in, 1 out]
        }
        n2969 = Merge Errors(w6970, w6967) -> (w6971:errorcluster)
      }
      frame "Test Channel 5E" {
        w7017 = T9 {"command"="", "data"=variant} ("element")
        w7039 = T9 {"command"="", "data"=variant} ("element")
        w7059 = 5  # DUT channel (1-10)
        n2970 = disable-structure shown="LOGGING==TRUE" {
          disable-tunnel: w7054 -> [w7087 _]
          frame condition #0 (active) {
            n2971 = Empty String/Path?(string/path=w7087) -> (empty?=w7089:bool)
            n2972 = Select(t="Quece timeout", s=w7089, f=w7087) -> (s? t:f=w7086:string)
            n2973 = call "string log (SubVI).vi"("state Name"=w7086) -> ()  [unwired: 9 in, 2 out]
          }
          frame condition #1 {
          }
        }
        n2974 = Bundle By Name(cluster=w7039, "command"="Apps.UI Update", "data"="E") -> (w7038:T9)
        n2975 = Bundle By Name(cluster=w7039, "command"="MEAS.AllRelaysOFF2") -> (w7031:T9)
        n2976 = Bundle By Name(cluster=w7039, "command"="Apps.WaitForEvent") -> (w7037:T9)
        n2977 = Build Array(w7038, w7031, w7037) -> (w7044:T9[])
        n2978 = for {
          tunnel: [w7077] -> w7050 mode=indexing
          shift-right: [w7078] -> w7052
          shift-left: w7045 -> [w7076]
          tunnel: w7044 -> [w7075] mode=indexing
          n2979 = Unbundle By Name(w7075) -> ("command"=w7074:string, "data"=w7073:variant)
          n2980 = call "App enquece.vi"("Priority Enquece"=TRUE, "command data"=w7073, "command"=w7074, "queue in"=w7076) -> ("error out"=w7077:errorcluster, "Queue out"=w7078:refnum<queue>)  [unwired: 6 in]
        }
        n2981 = call "FGV DRV stand.vi"() -> ("Sub-Test.DCV"=w7032:bool)  [unwired: 10 in, 1 out]
        n2982 = case shown="True" w7032 {
          tunnel: [w7063 w7065] -> w7034
          frame False {
            n2983 = Build Array("WaitFor", "MEAS.requestAC") -> (w7063:string[])
          }
          frame True {
            n2984 = Build Array("Test DRV 25", "Test DRV 26", "Test DRV 27", "Test DRV 28", "Test DRV 29", "WaitForE", "MEAS.requestAC") -> (w7065:string[])
          }
        }
        n2985 = Merge Errors(w7050) -> (w7043:errorcluster)
        n2986 = Reverse 1D Array(array=w7034) -> (reversed array=w7030:string[])
        n2987 = for {
          tunnel: w7030 -> [w7084] mode=indexing
          tunnel: [w7083] -> w7049 mode=indexing
          shift-right: [w7082] -> w7051
          shift-left: w7052 -> [w7085]
          tunnel: w7043 -> [w7081]
          n2988 = call "App enquece.vi"("Priority Enquece"=TRUE, "error in (no error)"=w7081, "command"=w7084, "queue in"=w7085) -> ("error out"=w7083:errorcluster, "Queue out"=w7082:refnum<queue>)  [unwired: 6 in]
        }
        n2989 = Initialize Array(FALSE ("element"), 6 ("dimension size")) -> (w7013:bool[])
        n2990 = Initialize Array(TRUE, 5 ("dimension size")) -> (w7012:bool[])
        n2991 = Merge Errors(w7049) -> (w7048:errorcluster)
        n2992 = Replace Array Subset(array=w7013, new element=w7012) -> (w7011:bool[])  [unwired: 1 in]
        n2993 = To Variant(anything=T3."mux10_1_channel5" ("mux10_1(x6)_encode")) -> (Variant=w7028:variant)
        n2994 = To Variant(anything=T4."demux1_10_channel5" ("demux1_10(x6)_encode")) -> (Variant=w7024:variant)
        n2995 = To Variant(anything=w7011) -> (Variant=w7020:variant)
        n2996 = Bundle By Name(cluster=w7017, "command"="MEAS.mux10-1", "data"=w7028) -> (w7023:T9)
        n2997 = Bundle By Name(cluster=w7017, "command"="MEAS.demux1-10", "data"=w7024) -> (w7022:T9)
        n2998 = Bundle By Name(cluster=w7017, "command"="MEAS.eMIC", "data"=w7020) -> (w7019:T9)
        n2999 = Build Array(w7023, w7022, w7019) -> (w7047:T9[])
        n3000 = Reverse 1D Array(array=w7047) -> (reversed array=w7046:T9[])
        n3001 = for {
          tunnel: w7046 -> [w7095] mode=indexing
          tunnel: [w7092] -> w7053 mode=indexing
          tunnel: w7048 -> [w7091]
          tunnel: w7051 -> [w7096]
          n3002 = Unbundle By Name(w7095) -> ("command"=w7094:string, "data"=w7093:variant)
          n3003 = call "App enquece.vi"("Priority Enquece"=TRUE, "error in (no error)"=w7091, "command data"=w7093, "command"=w7094, "queue in"=w7096) -> ("error out"=w7092:errorcluster)  [unwired: 5 in, 1 out]
        }
        n3004 = Merge Errors(w7056, w7053) -> (w7057:errorcluster)
      }
      frame "Test Channel 6E" {
        w7103 = T9 {"command"="", "data"=variant} ("element")
        w7125 = T9 {"command"="", "data"=variant} ("element")
        w7145 = 6  # DUT channel (1-10)
        n3005 = disable-structure shown="LOGGING==TRUE" {
          disable-tunnel: w7140 -> [w7173 _]
